vi "Get Device Inputs.vi"(8 "error in (no error)":errorcluster, 10 "Device Reference in":T8 format="%.0x", 11 "RT Data in":T1 {"Channels"."Voltage"."Ref"."Data Reference" format="%.0x"; "Channels"."Current"."Ref"."Data Reference" format="%.0x"; "Channels"."Read Volt"."Ref" format="%.0x"; "Channels"."Mode"."Ref" format="%.0x"}) -> (0 "error out":errorcluster, 2 "Device Ref out":T8 format="%.0x", 3 "RT Data out":T1 {"Channels"."Voltage"."Ref"."Data Reference" format="%.0x"; "Channels"."Current"."Ref"."Data Reference" format="%.0x"; "Channels"."Read Volt"."Ref" format="%.0x"; "Channels"."Mode"."Ref" format="%.0x"})   [LabVIEW 2011, in "Switch-DMM Custom Device.lvlib"]
uses:
  Switch-DMM Custom Device.lvlib
  <vilib>/NI Veristand/Custom Device API/Custom Device Item Ref.ctl
  Controls/RT Data.ctl
  Controls/Channels.ctl
  Controls/Single Channel.ctl
  <vilib>/NI Veristand/Custom Device API/Data Reference.ctl
  Controls/Block Channels.ctl
  <vilib>/NI Veristand/Custom Device API/Block Data Reference.ctl
  Controls/Communication.ctl
  Controls/Async Status.ctl
  Controls/Async State.ctl
  Controls/Async Command.ctl
  Controls/Async Events.ctl
  <vilib>/NI Veristand/Custom Device API/Data Access Type.ctl
  Controls/Globals.vi
  <vilib>/NI Veristand/Custom Device Tools/Custom Device Utility Library/NI VeriStand - Search for Item by Property.vi
  <vilib>/NI Veristand/Custom Device Tools/Custom Device Utility Library/Custom Device Utility Library.lvlib
  <vilib>/NI Veristand/Custom Device API/Custom Device API.lvlib
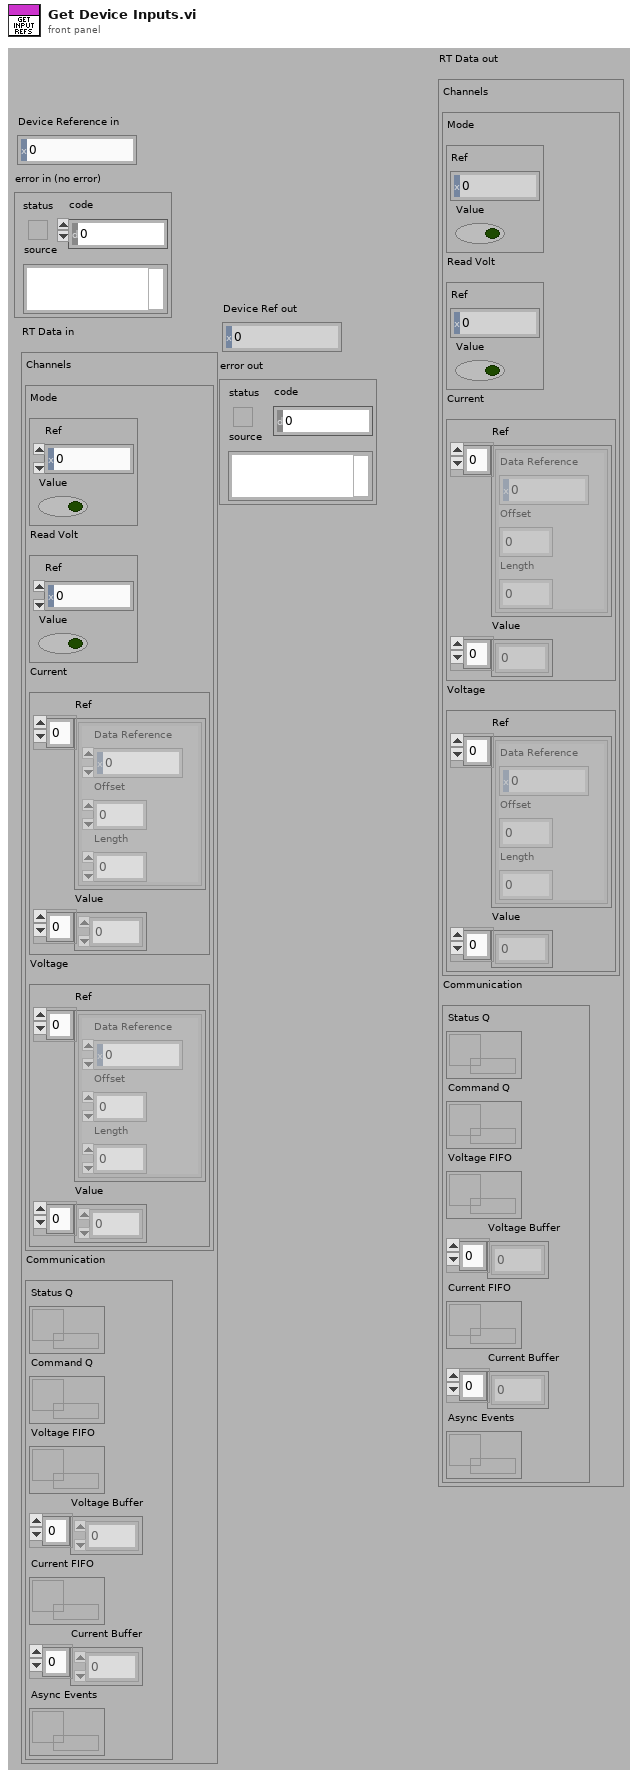
[diagram p1: front panel]
types:
  T1 = typedef "Switch-DMM Custom Device.lvlib/RT Data.ctl" = cluster{"Channels":T2, "Communication":T7}
  T2 = typedef "Switch-DMM Custom Device.lvlib/Channels.ctl" = cluster{"Mode":T3, "Read Volt":T3, "Current":T5, "Voltage":T5}
  T3 = typedef "Switch-DMM Custom Device.lvlib/Single Channel.ctl" = cluster{"Ref":T4, "Value":bool}
  T4 = typedef "Custom Device API.lvlib/Data Reference.ctl" = i32
  T5 = typedef "Switch-DMM Custom Device.lvlib/Block Channels.ctl" = cluster{"Ref":T6[], "Value":dbl[]}
  T6 = typedef "Custom Device API.lvlib/Block Data Reference.ctl" = cluster{"Data Reference":T4, "Offset":i32, "Length":i32}
  T7 = typedef "Switch-DMM Custom Device.lvlib/Communication.ctl" = cluster{"Status Q":refnum<queue>, "Command Q":refnum<queue>, "Voltage FIFO":refnum<k33>, "Voltage Buffer":dbl[], "Current FIFO":refnum<k33>, "Current Buffer":dbl[], "Async Events":refnum<queue>}
  T8 = typedef "Custom Device API.lvlib/Custom Device Item Ref.ctl" = u64
  T9 = typedef "Custom Device API.lvlib/Data Access Type.ctl" = enum16{"Read", "Write"}
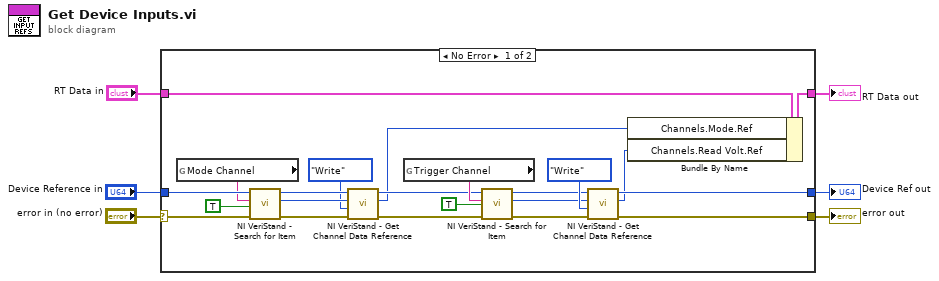
[diagram p0: block diagram]
diagram:
  n1 = case shown="No Error" "error in (no error)" {
    selector: "error in (no error)" -> [w25 w30]
    tunnel: "Device Reference in" -> [w28 w31]
    tunnel: [w12 w30] -> w4
    tunnel: [w11 w31] -> w3
    tunnel: [w8 w29] -> w2
    tunnel: "RT Data in" -> [w7 w29]
    frame No Error {
      n2 = global read "Globals.vi" "Mode Channel"() -> (w27:string)
      n3 = call-poly <vilib>:"NI VeriStand - Search for Item.vi"("error in"=w25, "Property Value"=TRUE, "Property Name"=w27, "Section Ref in"=w28) -> ("error out"=w22:errorcluster, "Item Ref"=w24:T8, "Section Ref out"=w23:T8)  [unwired: 4 in, 1 out]
      n4 = call <vilib>:"NI VeriStand - Get Channel Data Reference.vi"("error in (no error)"=w22, "Access"=Data_Access_Type."Write", "Channel Ref in"=w24, "Device Ref in"=w23) -> ("error out"=w13:errorcluster, "Channel Data Reference"=w10:T4, "Device Ref out"=w14:T8)  [unwired: 5 in]
      n5 = global read "Globals.vi" "Trigger Channel"() -> (w15:string)
      n6 = call-poly <vilib>:"NI VeriStand - Search for Item.vi"("error in"=w13, "Property Value"=TRUE, "Property Name"=w15, "Section Ref in"=w14) -> ("error out"=w19:errorcluster, "Item Ref"=w17:T8, "Section Ref out"=w18:T8)  [unwired: 4 in, 1 out]
      n7 = call <vilib>:"NI VeriStand - Get Channel Data Reference.vi"("error in (no error)"=w19, "Access"=Data_Access_Type."Write", "Channel Ref in"=w17, "Device Ref in"=w18) -> ("error out"=w12:errorcluster, "Channel Data Reference"=w9:T4, "Device Ref out"=w11:T8)  [unwired: 5 in]
      n8 = Bundle By Name(cluster=w7, "Channels.Mode.Ref"=w10, "Channels.Read Volt.Ref"=w9) -> (w8:T1)
    }
    frame Error {
    }
  }
  "Device Ref out" <- w3
  "error out" <- w4
  "RT Data out" <- w2
